vi "GDSProject_GetTargetFromProjectItem.vi"(8 "error in (no error)":errorcluster, 11 "ProjectItem in":refnum<vi>) -> (0 "error out":errorcluster, 3 "TargetItem out":refnum<vi>)   [LabVIEW 2020]
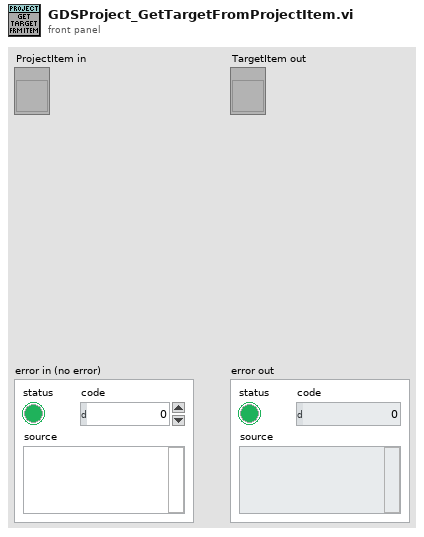
[diagram p1: front panel]
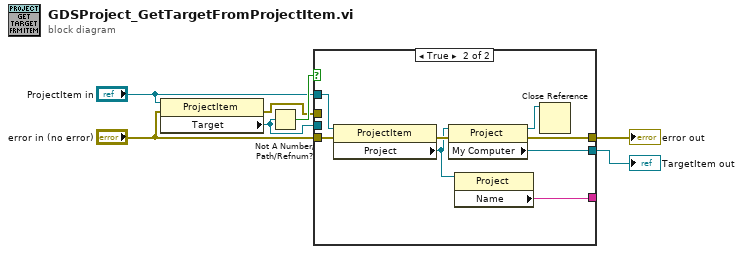
[diagram p0: block diagram]
diagram:
  n1 = property class="ProjectItem"(reference="ProjectItem in", error in="error in (no error)") -> (error out=w6:errorcluster, "Target"=w4:refnum<vi>)  [unwired: 1 out]
  n2 = Not A Number/Path/Refnum?(number/path/refnum=w4) -> (NaN/Path/Refnum?=w7:bool)
  n3 = case shown="True" w7 {
    tunnel: [w9 w16] -> w3
    tunnel: w4 -> [w9 _]
    tunnel: [w8 w17] -> w5
    tunnel: "error in (no error)" -> [_ w15]
    tunnel: w6 -> [w8 _]
    tunnel: "ProjectItem in" -> [_ w14]
    tunnel: [_ w10] -> _
    frame False {
    }
    frame True {
      n4 = property class="ProjectItem"(reference=w14, error in=w15) -> (error out=w13:errorcluster, "Project"=w11:refnum<vi>)  [unwired: 1 out]
      n5 = property class="Project"(reference=w11, error in=w13) -> (reference out=w12:refnum<vi>, error out=w17:errorcluster, "My Computer"=w16:refnum<vi>)
      n6 = property class="Project"(reference=w11) -> ("Name"=w10:string)  [unwired: 1 in, 2 out]
      n7 = Close Reference(reference=w12) -> ()  [unwired: 1 in, 1 out]
    }
  }
  "error out" <- w5
  "TargetItem out" <- w3
